vi "Read Channel Single Shot (Raw).vi"(8 "error in (no error)":errorcluster, 10 "ADC Channel Selection":T1, 11 "LINX-ADS1256 in":refnum<class "LINX-ADS1256.lvclass">) -> (0 "error out":errorcluster, 2 "ADC Raw":i32, 3 "LINX-ADS1256 out":refnum<class "LINX-ADS1256.lvclass">)   [LabVIEW 2020, in "LINX-ADS1256.lvclass"]
uses:
  LINX-ADS1256.lvclass
  Channel Selection.ctl
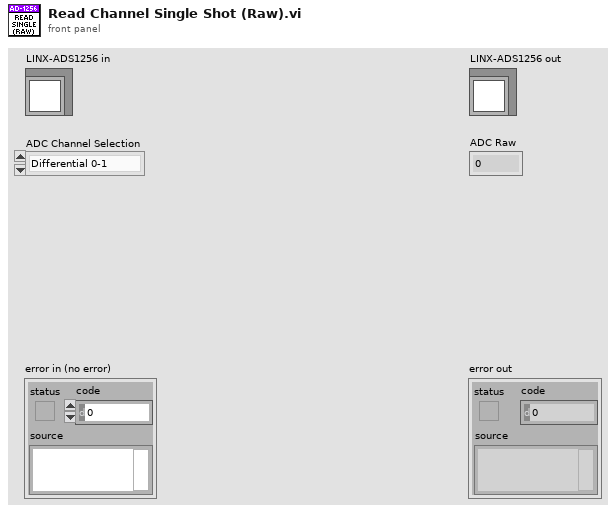
[diagram p1: front panel]
types:
  T1 = typedef "LINX-ADS1256.lvclass/Channel Selection.ctl" = enum16{"Differential 0-1", "Differential 2-3", "Differential 4-5", "Differential 6-7", "Single Ended 0", "Single Ended 1", "Single Ended 2", "Single Ended 3", "Single Ended 4", "Single Ended 5", "Single Ended 6", "Single Ended 7"}
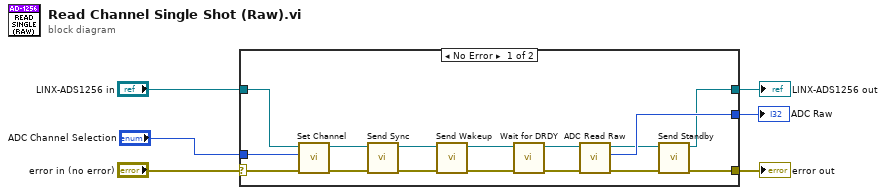
[diagram p0: block diagram]
diagram:
  n1 = case shown="No Error" "error in (no error)" {
    selector: "error in (no error)" -> [w14 w24]
    tunnel: [w7 w24] -> w5
    tunnel: [w8 w23] -> w3
    tunnel: "LINX-ADS1256 in" -> [w13 w23]
    tunnel: "ADC Channel Selection" -> [w12 _]
    tunnel: [w11 _] -> w1
    frame No Error {
      n2 = call "Set Channel.vi"("error in (no error)"=w14, "ADC Channel Selection"=w12, "LINX-ADS1256 in"=w13) -> ("error out"=w20:errorcluster, "LINX-ADS1256 out"=w19:refnum<class "LINX-ADS1256.lvclass">)  [unwired: 7 in]
      n3 = call "Send Sync.vi"("error in (no error)"=w20, "LINX-ADS1256 in"=w19) -> ("error out"=w18:errorcluster, "LINX-ADS1256 out"=w17:refnum<class "LINX-ADS1256.lvclass">)  [unwired: 8 in]
      n4 = call "Send Wakeup.vi"("error in (no error)"=w18, "LINX-ADS1256 in"=w17) -> ("error out"=w15:errorcluster, "LINX-ADS1256 out"=w16:refnum<class "LINX-ADS1256.lvclass">)  [unwired: 8 in]
      n5 = call "Wait for DRDY.vi"("error in (no error)"=w15, "LINX-ADS1256 in"=w16) -> ("error out"=w21:errorcluster, "LINX-ADS1256 out"=w22:refnum<class "LINX-ADS1256.lvclass">)  [unwired: 6 in, 2 out]
      n6 = call-dynamic "ADC Read Raw.vi"("error in (no error)"=w21, "LINX-ADS1256 in"=w22) -> ("error out"=w10:errorcluster, "ADC Raw"=w11:i32, "LINX-ADS1256 out"=w9:refnum<class "LINX-ADS1256.lvclass">)  [unwired: 7 in]
      n7 = call "Send Standby.vi"("error in (no error)"=w10, "LINX-ADS1256 in"=w9) -> ("error out"=w7:errorcluster, "LINX-ADS1256 out"=w8:refnum<class "LINX-ADS1256.lvclass">)  [unwired: 8 in]
    }
    frame Error {
    }
  }
  "error out" <- w5
  "LINX-ADS1256 out" <- w3
  "ADC Raw" <- w1
